vi "PipBoy_InitNotifyMenu.vi"(8 "error in (no error)":errorcluster, 11 "IconPath":path) -> (0 "error out":errorcluster, 2 "UE-NotifyMenu":refnum<event-registration>, 3 "NotifyIconRef":refnum<k24>, 5 "Context Menu":string[][](array[string]))   [LabVIEW 2014]
uses:
  <userlib>/NotifyIcon/TypeDefs/NotifyIcon User Event Ref.ctl
  System.Windows.Forms
  <userlib>/NotifyIcon/TypeDefs/NotifyIcon Events.ctl
  <userlib>/NotifyIcon/TypeDefs/NotifyIcon Event Registration Actions.ctl
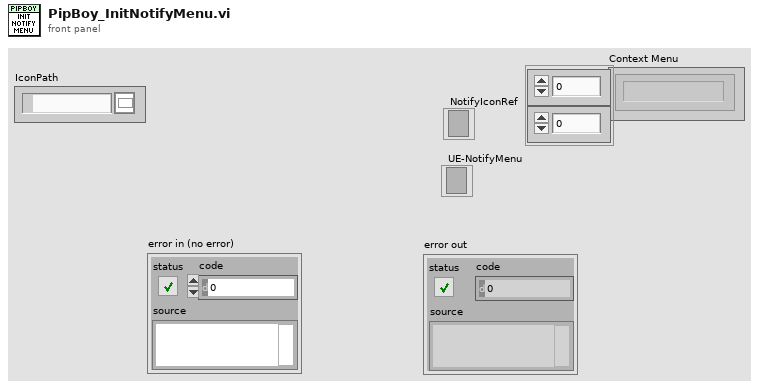
[diagram p1: front panel]
types:
  T1 = typedef "NotifyIcon Event Registration Actions.ctl" = enum16{"Initial Event Registration", "Add to Event Registration", "Destroy Events and Re-register"}
  T2 = typedef "NotifyIcon Events.ctl" = enum16{"BalloonTipClicked", "BalloonTipClosed", "BalloonTipShown", "Click", "Disposed", "DoubleClick", "MouseClick", "MouseDoubleClick", "MouseDown", "MouseMove", "MouseUp", "MenuItemClick", "MenuItemSelect"}
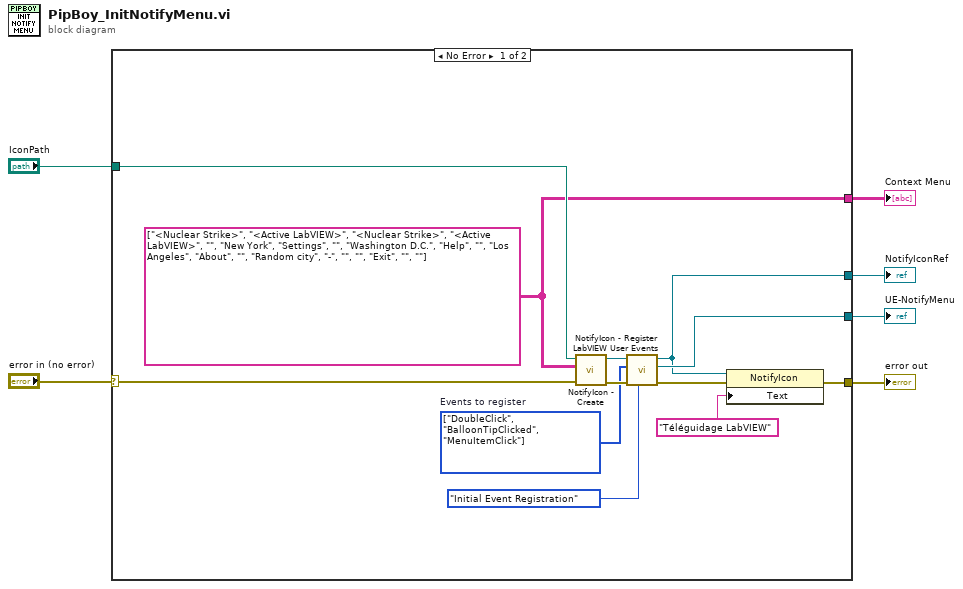
[diagram p0: block diagram]
diagram:
  n1 = case shown="No Error" "error in (no error)" {
    selector: "error in (no error)" -> [w14 w19]
    tunnel: [w8 w19] -> w5
    tunnel: [w13 _] -> w4
    tunnel: [w10 _] -> w3
    tunnel: "IconPath" -> [w12 _]
    tunnel: [w11 _] -> w1
    frame No Error {
      w11 = string[][] [["<Nuclear Strike>", "<Active LabVIEW>", "<Nuclear Strike>"], ["<Active LabVIEW>", "", "New York"], ["Settings", "", "Washington D.C."], ["Help", "", "Los Angeles"], ["About", "", "Random city"], ["-", "", ""], ["Exit", "", ""]] ("Context Menu (optional)")
      w16 = T2[] [enum."DoubleClick", enum."BalloonTipClicked", enum."MenuItemClick"] items=["BalloonTipClicked", "BalloonTipClosed", "BalloonTipShown", "Click", "Disposed", "DoubleClick", "MouseClick", "MouseDoubleClick", "MouseDown", "MouseMove", "MouseUp", "MenuItemClick", "MenuItemSelect"]  # Events to register
      n2 = call <userlib>:"NotifyIcon - Create.vi"("error in"=w14, "Context Menu (optional)"=w11, "Icon File Path"=w12) -> ("error out"=w17:errorcluster, "NotifyIcon reference"=w18:refnum<k24>)  [unwired: 7 in]
      n3 = call <userlib>:"NotifyIcon - Register LabVIEW User Events.vi"("Action"=NotifyIcon_Event_Registration_Actions."Initial Event Registration", "error in"=w17, "Events to register"=w16, "NotifyIcon reference in"=w18) -> ("error out"=w7:errorcluster, "Event Registration Refnum"=w13:refnum<event-registration>, "NotifyIcon reference out"=w10:refnum<k24>)  [unwired: 5 in]
      n4 = property class="NotifyIcon"(reference=w10, error in=w7, "Text"="Téléguidage LabVIEW") -> (error out=w8:errorcluster)  [unwired: 1 out]
    }
    frame Error {
    }
  }
  "error out" <- w5
  "UE-NotifyMenu" <- w4
  "NotifyIconRef" <- w3
  "Context Menu" <- w1
